vi "6. Read Nested Variables.vi"() -> ()   [LabVIEW 2017]
uses:
  6276dcbc-c98b-42be-a14e-8777d527878b.vi
  f718c417-406b-4765-8f4e-f4eec60edb5e.vi
  a3e32e02-708e-4059-a0d8-10937bb7013f.vi
  95f2009b-65fd-4f58-8c71-5d86384b1502.vi
  6e37e26f-aac1-44d7-bda5-9520715fecec.vi
  6276dcbc-c98b-42be-a14e-8777d527878b.vi/b09b9099-6be0-413b-8afc-4908471460c3.vi
  INI-Static-Variable-Support/_Support/FlagInstance-CSMINIVariable.vi
  f718c417-406b-4765-8f4e-f4eec60edb5e.vi/b09b9099-6be0-413b-8afc-4908471460c3.vi
  <userlib>/_NEVSTOP/Communicable State Machine(CSM)/addons/API-String-Arugments-Support/_Support/Concatenate Strings If not Empty_csm.vi
  95f2009b-65fd-4f58-8c71-5d86384b1502.vi/99de0c97-112a-4c86-9094-c187659127e1.vi
  <userlib>/_NEVSTOP/Communicable State Machine(CSM)/Utility/Build Error Cluster.vi
  6e37e26f-aac1-44d7-bda5-9520715fecec.vi/b09b9099-6be0-413b-8afc-4908471460c3.vi
  <userlib>/_NEVSTOP/Communicable State Machine(CSM)/_Support/ChangeFlag/ChangeFlag-Read.vi
  <userlib>/_NEVSTOP/Communicable State Machine(CSM)/_Support/ChangeFlag/ChangeFlagDB.vi
  <vilib>/Utility/Data Type/Get Type Information.vi
  <userlib>/_NEVSTOP/Communicable State Machine(CSM)/addons/API-String-Arugments-Support/_Support/Data To SingleElementsArray_csm.vi
  INI-Static-Variable-Support/_Support/Parse Used Session and Name.vi
  <userlib>/_NEVSTOP/Communicable State Machine(CSM)/addons/API-String-Arugments-Support/_Support/Data To API String Arguments.vi
  INI-Static-Variable-Support/_Support/INI-FGV(lvlibp).vi
  INI-Static-Variable-Support/_Support/Populate String with INI Variable.vi
  <userlib>/_NEVSTOP/Communicable State Machine(CSM)/addons/API-String-Arugments-Support/_Support/Convert API String Arguments to Data(variant).vi
  <userlib>/_NEVSTOP/Communicable State Machine(CSM)/addons/API-String-Arugments-Support/_Support/SingleElementsArray To Data_csm.vi
  INI-Static-Variable-Support/INI-Static-Variable-Support.lvlib
panel:
  out "from key 2":string
  out "from section":cluster{"addr":string}
  out "${rt.addr} 2":string
  out "rt.cluster2":cluster{"select":string, "addr":string}
  out "${file.path}":string
  out "case1.addr":string
  out "case2.addr":string
  out "rt.cluster":cluster{"select":string, "addr":string}
  out "${rt.addr}":string
  out "${network.url}":string
  out "${network.url}":string
  out "network.cluster":cluster{"url":string, "host":string}
  out "${network.url}":string
  out "${network.host}":string
  # "5. One common scenario for nested variable\nBuild saving path for file loaction"
  # "4. Use rt.select as a pointer to section.\nChange rt.select, will make rt.addr different."
  # "3. Nested variable in multiple section"
  # "2. Nested variable in one section"
  # "#CSM-Example overview"
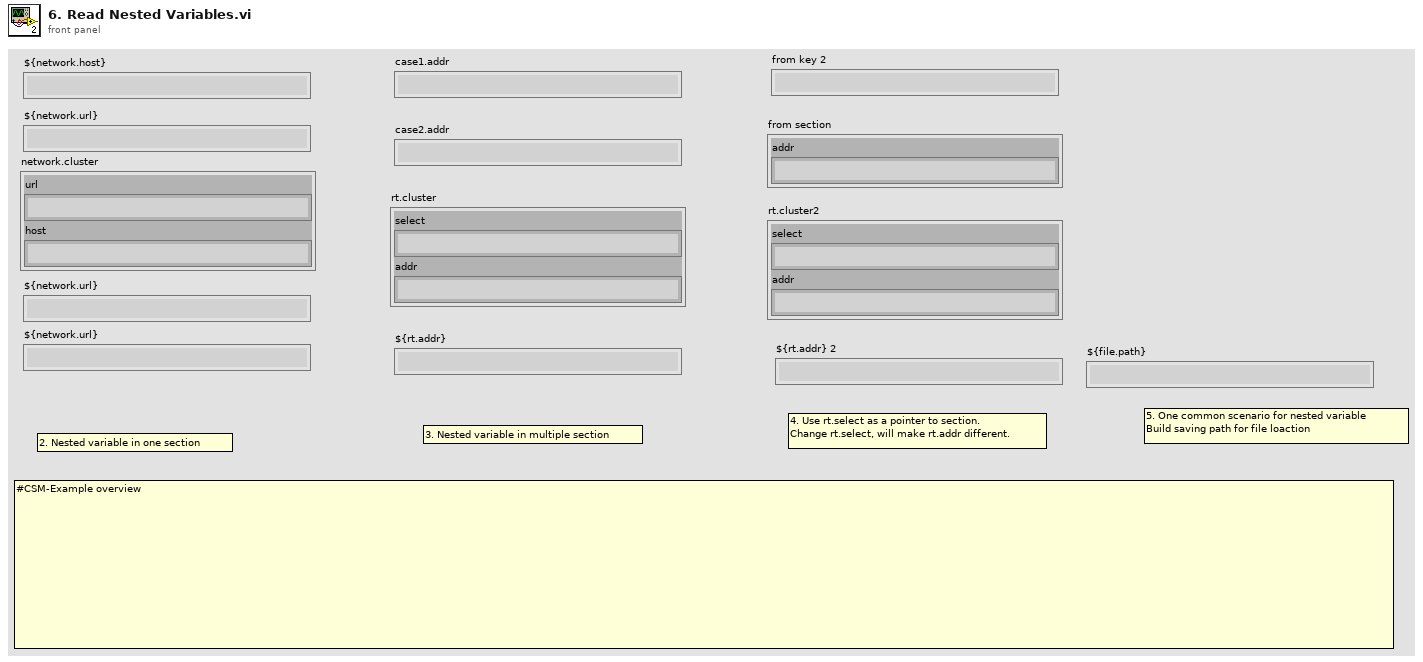
[diagram p1: front panel]
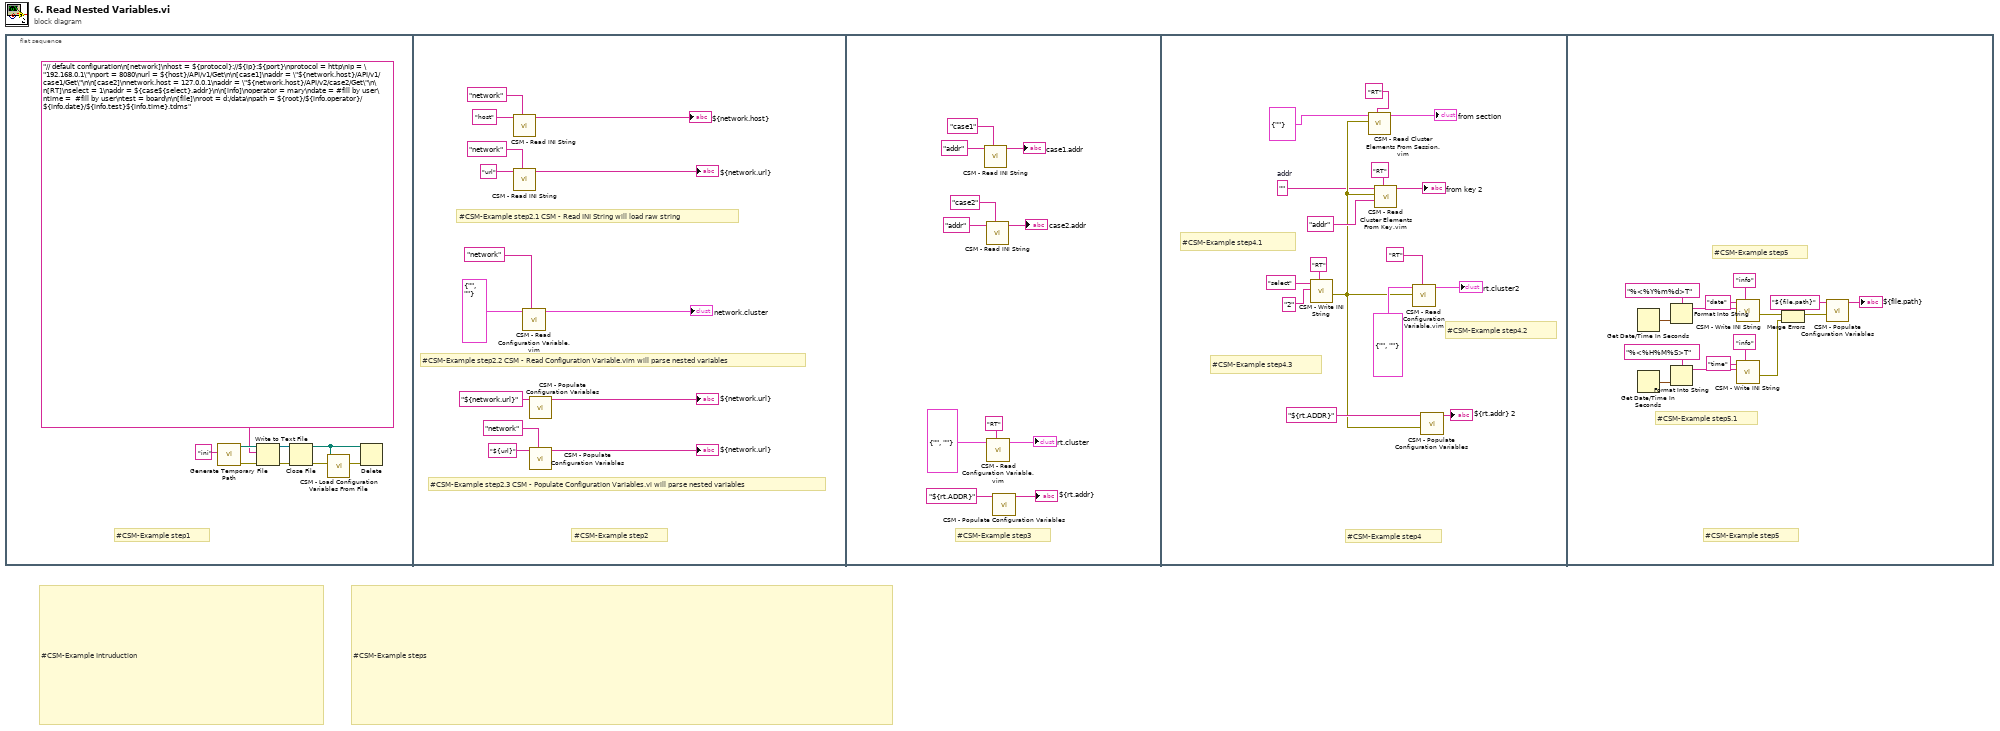
[diagram p0: block diagram]
diagram:
  # "#CSM-Example steps"
  # "#CSM-Example Intruduction"
  n1 = flat-sequence {
    frame #0 {
      # "#CSM-Example step1"
      n2 = call <vilib>:"Generate Temporary File Path.vi"("Temporary File Extension (tmp)"="ini") -> ("error out"=w9:errorcluster, "Unique Temporary File Path"=w6:path)  [unwired: 9 in]
      n3 = Write to Text File(file (use dialog)=w6, text="// default configuration\n[network]\nhost = ${protocol}://${ip}:${port}\nprotocol = http\nip = \"192.168.0.1\"\nport = 8080\nurl = ${host}/API/v1/Get\n\n[case1]\naddr = \"${network.host}/API/v1/case1/Get\"\n\n[case2]\nnetwork.host = 127.0.0.1\naddr = \"${network.host}/API/v2/case2/Get\"\n\n[RT]\nselect = 1\naddr = ${case${select}.addr}\n\n[info]\noperator = mary\ndate = #fill by user\ntime =  #fill by user\ntest = board\n\n[file]\nroot = d:/data\npath = ${root}/${info.operator}/${info.date}/${info.test}${info.time}.tdms", error in=w9) -> (refnum out=w5:refnum<file>, error out=w7:errorcluster)  [unwired: 1 in, 1 out]
      n4 = Close File(refnum=w5, error in=w7) -> (path=w1:path, error out=w4:errorcluster)
      n5 = call "CSM - Load Configuration Variables From File.vi"("error in (no error)"=w4, "Configuration Path"=w1) -> ("error out"=w2:errorcluster)  [unwired: 7 in]
      n6 = Delete(path (use dialog)=w1, error in=w2) -> ()  [unwired: 3 in, 3 out]
    }
    frame #1 {
      # "#CSM-Example step2"
      # "#CSM-Example step2.3 CSM - Populate Configuration Variables.vi will parse nested variables"
      # "#CSM-Example step2.2 CSM - Read Configuration Variable.vim will parse nested variables"
      # "#CSM-Example step2.1 CSM - Read INI String will load raw string"
      n7 = call "CSM - Read INI String.vi"("Section Name (\"\" as Default)"="network" ("Section Name(\"\" as Default)"), "Variable Name"="host" ("String in")) -> ("Value"=→"${network.host}":string)  [unwired: 5 in, 2 out]
      n8 = call "CSM - Read INI String.vi"("Section Name (\"\" as Default)"="network" ("Section Name(\"\" as Default)"), "Variable Name"="url" ("String in")) -> ("Value"=→"${network.url}":string)  [unwired: 5 in, 2 out]
      n9 = call "CSM - Read Configuration Variable.vim"("Section Name (\"\" as Default)"="network" ("Section Name(\"\" as Default)"), "Configuration Prototype (Cluster Prefered)"=cluster{"url":string, "host":string} {"url"="", "host"=""}) -> ("Configuration"=→"network.cluster":cluster{"url":string, "host":string})  [unwired: 6 in, 1 out]
      n10 = call "CSM - Populate Configuration Variables.vi"("String with INI-Variable"="${network.url}" ("String in")) -> ("String"=→"${network.url}":string)  [unwired: 7 in, 1 out]
      n11 = call "CSM - Populate Configuration Variables.vi"("Section Name (\"\" as Default)"="network" ("Section Name(\"\" as Default)"), "String with INI-Variable"="${url}" ("String in")) -> ("String"=→"${network.url}":string)  [unwired: 6 in, 1 out]
    }
    frame #2 {
      # "#CSM-Example step3"
      n12 = call "CSM - Read INI String.vi"("Section Name (\"\" as Default)"="case1" ("Section Name(\"\" as Default)"), "Variable Name"="addr" ("String in")) -> ("Value"=→"case1.addr":string)  [unwired: 5 in, 2 out]
      n13 = call "CSM - Read INI String.vi"("Section Name (\"\" as Default)"="case2" ("Section Name(\"\" as Default)"), "Variable Name"="addr" ("String in")) -> ("Value"=→"case2.addr":string)  [unwired: 5 in, 2 out]
      n14 = call "CSM - Read Configuration Variable.vim"("Section Name (\"\" as Default)"="RT" ("Section Name(\"\" as Default)"), "Configuration Prototype (Cluster Prefered)"=cluster{"select":string, "addr":string} {"select"="", "addr"=""}) -> ("Configuration"=→"rt.cluster":cluster{"select":string, "addr":string})  [unwired: 6 in, 1 out]
      n15 = call "CSM - Populate Configuration Variables.vi"("String with INI-Variable"="${rt.ADDR}" ("String in")) -> ("String"=→"${rt.addr}":string)  [unwired: 7 in, 1 out]
    }
    frame #3 {
      w35 = ""  # addr
      # "#CSM-Example step4.3"
      # "#CSM-Example step4.2"
      # "#CSM-Example step4.1"
      # "#CSM-Example step4"
      n16 = call "CSM - Write INI String.vi"("Section Name (\"\" as Default)"="RT" ("Section Name(\"\" as Default)"), "Value"="2" (">> Variable Name >>"), "Key"="select" (">> Variable Name >>")) -> ("error out"=w36:errorcluster)  [unwired: 5 in, 1 out]
      n17 = call "CSM - Read Cluster Elements From Session.vim"("Section Name (\"\" as Default)"="RT" ("Section Name(\"\" as Default)"), "error in (no error)"=w36, "Cluster"=cluster{"addr":string} {"addr"=""}) -> ("Cluster out"=→"from section":cluster{"addr":string})  [unwired: 5 in, 1 out]
      n18 = call "CSM - Read Cluster Elements From Key.vim"("Section Name (\"\" as Default)"="RT" ("Section Name(\"\" as Default)"), "Key"="addr" ("Section Name(\"\" as Default)"), "error in (no error)"=w36, "Cluster"=w35) -> ("Cluster out"=→"from key 2":string)  [unwired: 3 in, 2 out]
      n19 = call "CSM - Read Configuration Variable.vim"("Section Name (\"\" as Default)"="RT" ("Section Name(\"\" as Default)"), "error in (no error)"=w36, "Configuration Prototype (Cluster Prefered)"=cluster{"select":string, "addr":string} {"select"="", "addr"=""}) -> ("Configuration"=→"rt.cluster2":cluster{"select":string, "addr":string})  [unwired: 5 in, 1 out]
      n20 = call "CSM - Populate Configuration Variables.vi"("error in (no error)"=w36, "String with INI-Variable"="${rt.ADDR}" ("String in")) -> ("String"=→"${rt.addr} 2":string)  [unwired: 6 in, 1 out]
    }
    frame #4 {
      # "#CSM-Example step5.1"
      # "#CSM-Example step5"
      # "#CSM-Example step5"
      n21 = Get Date/Time In Seconds() -> (seconds since 1Jan1904=w65:timestamp)
      n22 = Get Date/Time In Seconds() -> (seconds since 1Jan1904=w53:timestamp)
      n23 = Format Into String(format string="%<%Y%m%d>T", w65) -> (resulting string=w63:string)  [unwired: 2 in, 1 out]
      n24 = Format Into String(format string="%<%H%M%S>T", w53) -> (resulting string=w55:string)  [unwired: 2 in, 1 out]
      n25 = call "CSM - Write INI String.vi"("Section Name (\"\" as Default)"="info" ("Section Name(\"\" as Default)"), "Value"=w63, "Key"="date" (">> Variable Name >>")) -> ("error out"=w59:errorcluster)  [unwired: 5 in, 1 out]
      n26 = call "CSM - Write INI String.vi"("Section Name (\"\" as Default)"="info" ("Section Name(\"\" as Default)"), "Value"=w55, "Key"="time" (">> Variable Name >>")) -> ("error out"=w51:errorcluster)  [unwired: 5 in, 1 out]
      n27 = Merge Errors(w59, w51) -> (w52:errorcluster)
      n28 = call "CSM - Populate Configuration Variables.vi"("error in (no error)"=w52, "String with INI-Variable"="${file.path}" ("String in")) -> ("String"=→"${file.path}":string)  [unwired: 6 in, 1 out]
    }
  }
